vi "Write Waveform to Database.vi"(6 "Field":string="PhaseNoiseID", 7 "Table":string="APA.PhaseNoise_Data", 8 "error in (no error)":errorcluster, 9 "Array":sgl[][](array[numeric]), 10 "FreqID":i32, 11 "conninfo":path) -> (0 "error out":errorcluster)   [LabVIEW 2017]
uses:
  <vilib>/addons/database/Connection.llb/DB Tools Open Connec (Path).vi
  <vilib>/addons/database/NI_Database_API.lvlib
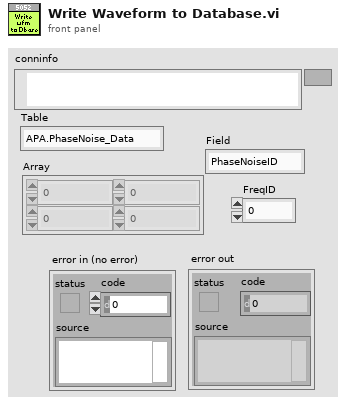
[diagram p1: front panel]
types:
  T1 = typedef "NI_Database_API.lvlib/Conn ObjectReference.ctl" = refnum<k1>
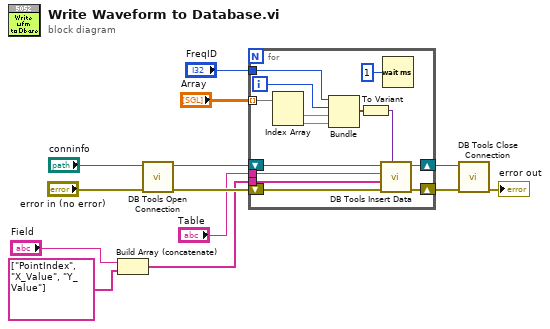
[diagram p0: block diagram]
diagram:
  n1 = Build Array (concatenate)("Field", string[] ["PointIndex", "X_Value", "Y_Value"] ("columns")) -> (w1:string[])
  n2 = call-poly <vilib>:"DB Tools Open Connection.vi"("error in (no error)"="error in (no error)", "connection information"="conninfo") -> ("error out"=w11:errorcluster, "connection reference"=w10:T1)  [unwired: 6 in]
  n3 = for {
    tunnel: "Table" -> [w25]
    tunnel: w1 -> [w24]
    tunnel: "Array" -> [w21] mode=indexing
    tunnel: "FreqID" -> [w23]
    shift-right: [w15] -> w5
    shift-left: w10 -> [w26]
    shift-right: [w16] -> w6
    shift-left: w11 -> [w27]
    i -> [w22]
    n4 = Index Array(array=w21) -> (element #1=w20:sgl, element #2=w19:sgl)  [unwired: 2 in]
    n5 = Bundle("FreqID"=w23, w22, w20, w19) -> (w18:cluster{"FreqID":i32, i32, sgl, sgl})  [unwired: 1 in]
    n6 = To Variant(anything=w18) -> (Variant=w17:variant)
    n7 = call <vilib>:"DB Tools Insert Data.vi"("data"=w17, "error in (no error)"=w27, "columns"=w24, "table"=w25, "connection reference"=w26) -> ("error out"=w16:errorcluster, "connection reference out"=w15:T1)  [unwired: 5 in]
    n8 = Wait (ms)(milliseconds to wait=u32 1) -> ()  [unwired: 1 out]
  }
  n9 = call <vilib>:"DB Tools Close Connection.vi"("error in (no error)"=w6, "connection reference"=w5) -> ("error out"=→"error out":errorcluster)  [unwired: 5 in]
